vi "Move to Array of Points.vi"() -> ()   [LabVIEW 2017]
uses:
  040-typeDefs/Position.ctl
panel:
  in  "stop":bool
  in  "Array":T1[](array[typedef])=[{"X Pos"=0.0, "Y Pos"=1000.0, "Bearing"=0.0}, {"X Pos"=1000.0, "Y Pos"=1000.0, "Bearing"=0.0}]
  out "Final X, Y, BEARING":cluster{dbl, dbl, dbl}
  in  "Initial X, Y, BEARING":cluster{dbl, dbl, dbl}
  in  "Max Speed":dbl=3.0
  in  "threshold":dbl=10.0
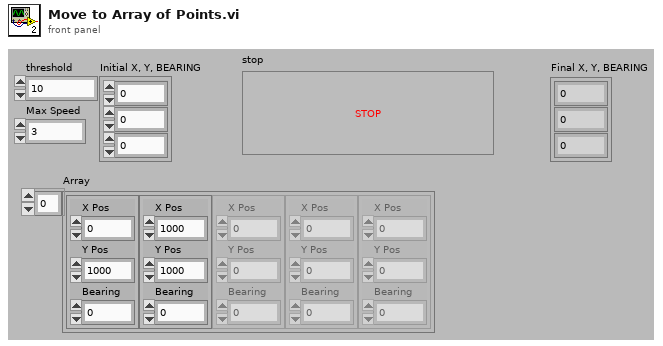
[diagram p1: front panel]
types:
  T1 = typedef "Position.ctl" = cluster{"X Pos":dbl, "Y Pos":dbl, "Bearing":dbl}
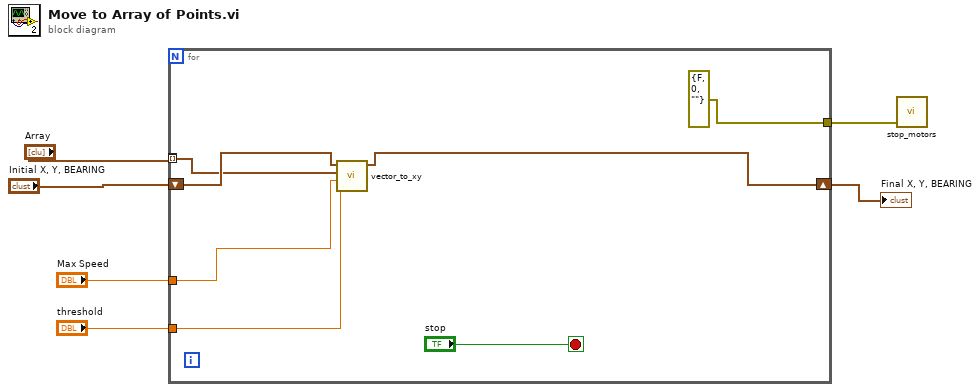
[diagram p0: block diagram]
diagram:
  n1 = for {
    tunnel: "Max Speed" -> [w12]
    tunnel: "threshold" -> [w11]
    shift-right: [w10] -> w3
    shift-left: "Initial X, Y, BEARING" -> [w13]
    tunnel: [w9] -> _ mode=indexing
    tunnel: "Array" -> [w9] mode=indexing
    tunnel: [errorcluster {"status"=FALSE, "code"=0, "source"=""} ("error constant")] -> w1
    stop <- "stop" stop-if-true
    n2 = call "vector_to_xy.vi"("threshold"=w11, "Max Speed"=w12, 10:w9, "Initial X, Y, BEARING"=w13) -> ("Final X, Y, BEARING"=w10:cluster{dbl, dbl, dbl})  [unwired: 7 in]
  }
  "Final X, Y, BEARING" <- w3
  n3 = call "stop_motors.vi"("error in (no error)"=w1) -> ()  [unwired: 4 in, 1 out]
